vi "DepthSense Create.vi"(8 "Denoise?":bool=TRUE, 9 "Close Mode?":bool=TRUE, 10 "Framerate":enum32{"25", "30", "50", "60"}(ring), 11 "Confidence":i32) -> (0 "error out":errorcluster, 2 "DepthSense Status":T1={"Camera Version"="", "Image Height"=0, "Image Width"=0, "Minimum Framerate"=0, "Maximum Framerate"=0, "Framerate"=25, "Close Mode"=FALSE, "Denoising"=FALSE, "Leakage Algorithm"=FALSE, "Anti-Aliasing"=FALSE, "Camera Status"=-2, "API Version"="", "Light Intensity"=100, "Confidence Threshold"=100, "Range"=0.0}, 3 "callbacks":cluster{"References":T2, "References":T2})   [LabVIEW 2011]
uses:
  FunctionPointerProxy/LabVIEW/t_CallbackReferences.ctl
  C:/Users/Behavior Room/Desktop/Kinect Mouse/DepthSense/FunctionPointerProxy/FunctionPointerProxy/bin/Release/FunctionPointerProxy.dll
  FunctionPointerProxy/FunctionPointerProxy/bin/Release/FunctionPointerProxy.dll
  <vilib>/vision/Image Controls.llb/IMAQ Image.ctl
  IT WORKS SO SUCK IT/DepthSense Global Status.vi
  <userlib>/libOptrima-2-3/libOptrima-2-3.lvlib
  Program Files (x86)/SoftKinetic/OptrimaSDK/lib/libOptrima-2-3.dll
panel:
  in  "DepthSense Indicator":T3={"Camera Version"="", "Image Height"=0, "Image Width"=0, "Minimum Framerate"=0, "Maximum Framerate"=0, "Framerate"=25, "Close Mode"=FALSE, "Denoising"=FALSE, "Leakage Algorithm"=FALSE, "Anti-Aliasing"=FALSE, "Camera Status"=-2, "API Version"="", "Light Intensity"=100, "Confidence Threshold"=100, "Range"=0.0}
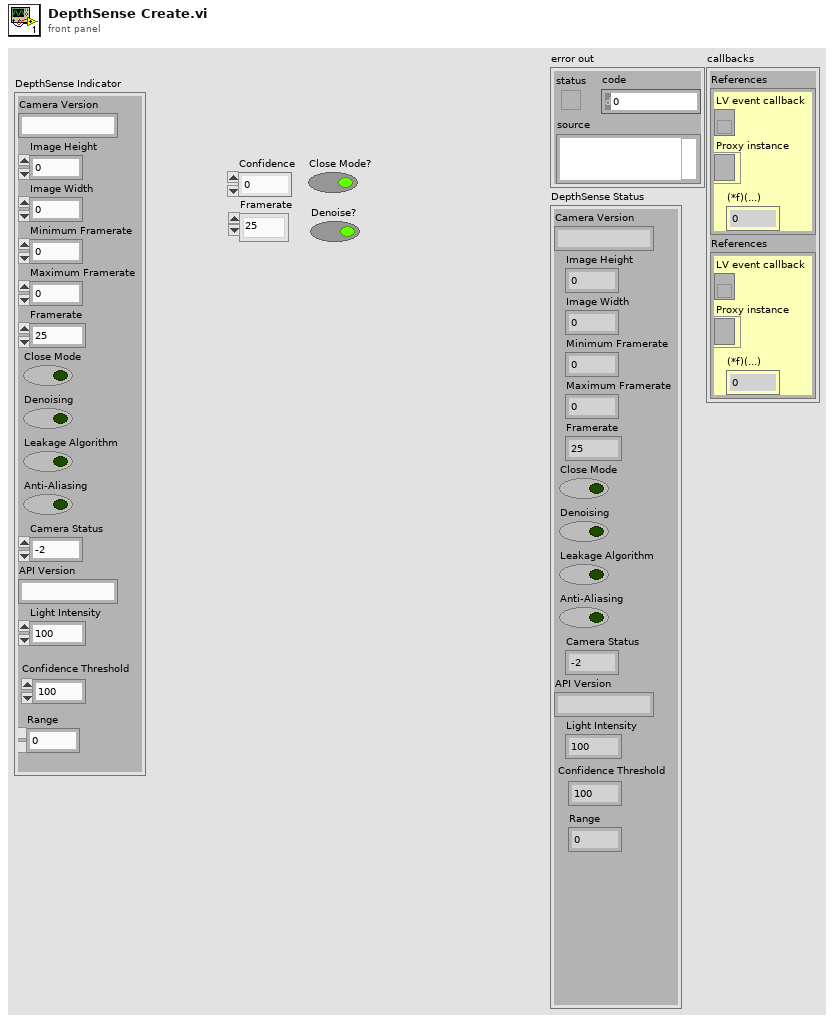
[diagram p1: front panel]
types:
  T1 = cluster{"Camera Version":string, "Image Height":i32, "Image Width":i32, "Minimum Framerate":i32, "Maximum Framerate":i32, "Framerate":i32, "Close Mode":bool, "Denoising":bool, "Leakage Algorithm":bool, "Anti-Aliasing":bool, "Camera Status":i32, "API Version":string, "Light Intensity":i32, "Confidence Threshold":u16, "Range":sgl}
  T2 = typedef "t_CallbackReferences.ctl" = cluster{"LV event callback ":refnum<k27>, "Proxy instance":refnum<k24>, "(*f)(...)":i32}
  T3 = cluster{"Camera Version":string, "Image Height":i32, "Image Width":i32, "Minimum Framerate":i32, "Maximum Framerate":i32, "Framerate":i32, "Close Mode":bool, "Denoising":bool, "Leakage Algorithm":bool, "Anti-Aliasing":bool, "Camera Status":i32, "API Version":string, "Light Intensity":i32, "Confidence Threshold":u16, "Range":dbl}
  T4 = typedef "IMAQ Image.ctl" = refnum<image>
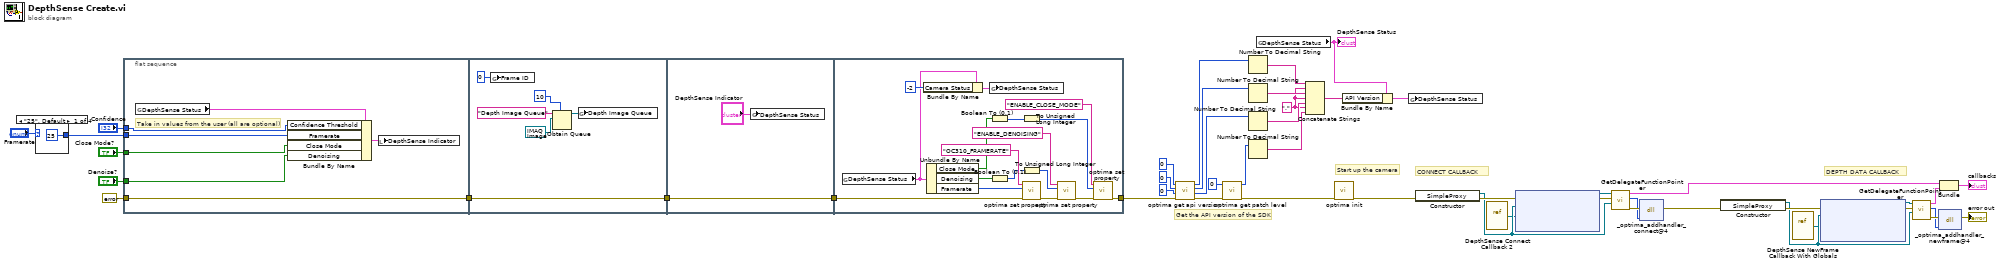
[diagram p0: block diagram]
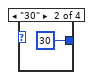
[diagram p2: hidden frame]
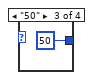
[diagram p3: hidden frame]
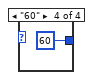
[diagram p4: hidden frame]
diagram:
  w34 = "."
  # "Get the API version of the SDK"
  # "Start up the camera"
  # "DEPTH DATA CALLBACK"
  # "CONNECT CALLBACK"
  n1 = case shown="\"25\", Default" "Framerate" {
    tunnel: [25 30 50 60] -> w2
    frame "25", Default {
    }
    frame "30" {
    }
    frame "50" {
    }
    frame "60" {
    }
  }
  n2 = flat-sequence {
    tunnel: errorcluster {"status"=FALSE, "code"=0, "source"=""} ("error in (no error)") -> [w59]
    tunnel: [w59] -> w9
    tunnel: "Close Mode?" -> [w57]
    tunnel: "Denoise?" -> [w56]
    tunnel: w2 -> [w55]
    tunnel: "Confidence" -> [w54]
    tunnel: [w65] -> w10
    tunnel: w9 -> [w65]
    tunnel: [w67] -> w48
    tunnel: w10 -> [w67]
    tunnel: [w82] -> w15
    tunnel: w48 -> [w76]
    frame #0 {
      # "Take in values from the user (all are optional)"
      n3 = global read "DepthSense Global Status.vi" "DepthSense Status"() -> (w58:T1)
      n4 = Bundle By Name(cluster=w58, "Confidence Threshold"=w54, "Framerate"=w55, "Close Mode"=w57, "Denoising"=w56) -> (w53:T1)
      n5 = local write "DepthSense Indicator"(w53) -> ()
    }
    frame #1 {
      n6 = global write "DepthSense Global Status.vi" "Frame ID"(0 ("Frame ID")) -> ()
      n7 = Obtain Queue(max queue size (-1, unlimited)=10, name (unnamed)="Depth Image Queue", element data type=T4 refnum ("New Image")) -> (queue out=w62:refnum<queue>)  [unwired: 2 in, 2 out]
      n8 = global write "DepthSense Global Status.vi" "Depth Image Queue"(w62) -> ()
    }
    frame #2 {
      n9 = global write "DepthSense Global Status.vi" "DepthSense Status"("DepthSense Indicator") -> ()
    }
    frame #3 {
      n10 = global read "DepthSense Global Status.vi" "DepthSense Status"() -> (w75:T1)
      n11 = Bundle By Name(cluster=w75, "Camera Status"=-2) -> (w84:T1)
      n12 = Unbundle By Name(w75) -> ("Close Mode"=w73:bool, "Denoising"=w71:bool, "Framerate"=w68:i32)
      n13 = global write "DepthSense Global Status.vi" "DepthSense Status"(w84) -> ()
      n14 = Boolean To (0,1)(Boolean=w73) -> (0, 1=w74:i16)
      n15 = Boolean To (0,1)(Boolean=w71) -> (0, 1=w72:i16)
      n16 = To Unsigned Long Integer(number=w74) -> (unsigned 32bit integer=w69:u32)
      n17 = To Unsigned Long Integer(number=w72) -> (unsigned 32bit integer=w70:u32)
      n18 = call <userlib>:"optrima set property.vi"("error in (no error)"=w76, "value"=w68, "name"="OC310_FRAMERATE") -> ("error out"=w79:errorcluster)  [unwired: 7 in, 1 out]
      n19 = call <userlib>:"optrima set property.vi"("error in (no error)"=w79, "value"=w70, "name"="ENABLE_DENOISING") -> ("error out"=w78:errorcluster)  [unwired: 7 in, 1 out]
      n20 = call <userlib>:"optrima set property.vi"("error in (no error)"=w78, "value"=w69, "name"="ENABLE_CLOSE_MODE") -> ("error out"=w82:errorcluster)  [unwired: 7 in, 1 out]
    }
  }
  n21 = call <userlib>:"optrima get api version.vi"("error in (no error)"=w15, "minor"=u32 0, "major"=u32 0, "release"=u32 0) -> ("error out"=w47:errorcluster, "minor out"=w44:u32, "major out"=w45:u32, "release out"=w46:u32)  [unwired: 4 in]
  n22 = call <userlib>:"optrima get patch level.vi"("error in (no error)"=w47, "patch"=u32 0) -> ("error out"=w14:errorcluster, "patch out"=w43:u32)  [unwired: 8 in]
  n23 = Number To Decimal String(number=w46) -> (decimal integer string=w42:string)  [unwired: 1 in]
  n24 = Number To Decimal String(number=w45) -> (decimal integer string=w37:string)  [unwired: 1 in]
  n25 = Number To Decimal String(number=w44) -> (decimal integer string=w36:string)  [unwired: 1 in]
  n26 = Number To Decimal String(number=w43) -> (decimal integer string=w35:string)  [unwired: 1 in]
  n27 = global read "DepthSense Global Status.vi" "DepthSense Status"() -> (w7:T1)
  "DepthSense Status" <- w7
  n28 = Concatenate Strings(w42, w34, w37, w34, w36, w34, w35) -> (w27:string)
  n29 = call <userlib>:"optrima init.vi"("error in (no error)"=w14) -> ("error out"=w13:errorcluster)  [unwired: 10 in]
  n30 = Bundle By Name(cluster=w7, "API Version"=w27) -> (w17:T1)
  n31 = global write "DepthSense Global Status.vi" "DepthSense Status"(w17) -> ()
  n32 = constructor class="SimpleProxy"(error in=w13) -> (reference out=w30:refnum<k24>, error out=w33:errorcluster)  [unwired: 2 in, 1 out]
  n33 = vi-ref "DepthSense Connect Callback 2.vi"() -> ("vi reference"=w26:refnum<vi>)
  n34 = node(w33, w30, w26) -> (w32:refnum<k27>, w31:errorcluster)  [unwired: 2 in]
  n35 = call "GetDelegateFunctionPointer.vi"("target class"=w30, "error in (no error)"=w31, "event callback refnum"=w32) -> ("error out"=w29:errorcluster, "(*f)(...)"=w28:i32, "References"=w12:T2)  [unwired: 6 in]
  n36 = dll-call lib="C:/Program Files (x86)/SoftKinetic/OptrimaSDK/lib/libOptrima-2-3.dll" fn="_optrima_addhandler_connect@4"(error in=w29, "handlerfunc"=w28) -> (error out=w18:errorcluster)  [unwired: 4 in, 1 out]
  n37 = constructor class="SimpleProxy"(error in=w18) -> (reference out=w24:refnum<k24>, error out=w25:errorcluster)  [unwired: 2 in, 1 out]
  n38 = vi-ref "DepthSense NewFrame Callback With Globals.vi"() -> ("vi reference"=w19:refnum<vi>)
  n39 = node(w25, w24, w19) -> (w22:refnum<k27>, w23:errorcluster)  [unwired: 2 in]
  n40 = call "GetDelegateFunctionPointer.vi"("target class"=w24, "error in (no error)"=w23, "event callback refnum"=w22) -> ("error out"=w21:errorcluster, "(*f)(...)"=w20:i32, "References"=w11:T2)  [unwired: 6 in]
  n41 = dll-call lib="C:/Program Files (x86)/SoftKinetic/OptrimaSDK/lib/libOptrima-2-3.dll" fn="_optrima_addhandler_newframe@4"(error in=w21, "handlerfunc"=w20) -> (error out=→"error out":errorcluster)  [unwired: 4 in, 1 out]
  n42 = Bundle("References"=w12, "References"=w11) -> (→"callbacks":cluster{"References":T2, "References":T2})  [unwired: 1 in]
